vi "ArrayMin.vi"(9 "Array":dbl[](array[numeric])) -> (1 "min":dbl)   [LabVIEW 2016]
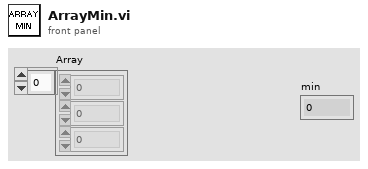
[diagram p1: front panel]
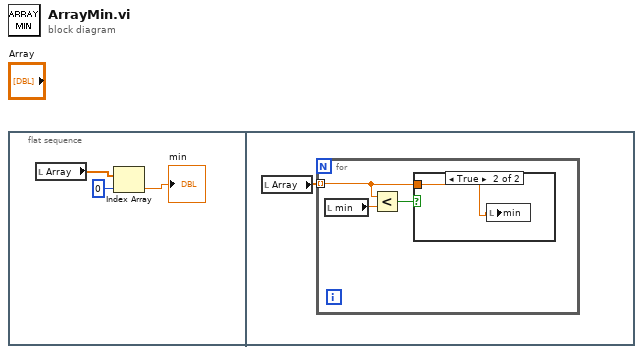
[diagram p0: block diagram]
diagram:
  n1 = flat-sequence {
    frame #0 {
      n2 = local read "Array"() -> (w2:dbl[])
      n3 = Index Array(array=w2, index=0) -> (element=→"min":dbl)
    }
    frame #1 {
      n4 = local read "Array"() -> (w4:dbl[])
      n5 = for {
        tunnel: w4 -> [w5] mode=indexing
        n6 = local read "min"() -> (w6:dbl)
        n7 = Less?(x=w5, y=w6) -> (x < y?=w7:bool)
        n8 = case shown="True" w7 {
          tunnel: w5 -> [_ w8]
          frame False {
          }
          frame True {
            n9 = local write "min"(w8) -> ()
          }
        }
      }
    }
  }
